vi "MenuSelection(User).vi"(6 "User events":T8, 7 "Clipboard":refnum<vi>, 8 "error in":errorcluster {"code" min=0 max=0}, 10 "ItemTag":string, 11 "Data in":T1={"Class"={"Ants"=refnum, "Layer"=refnum, "Templates"=refnum, "Icon"=refnum, "Glyph"=refnum, "Settings"=refnum, "Tools"=refnum, "History"=refnum}, "Ref"={"Add Layer"=refnum, "Remove Layer"=refnum, "Line Text"=[], "Body Text Spec"=refnum, "DNL_Font"=refnum, "glyph path str"=refnum, "templates path str"=refnum, "Arrow Up"=refnum, "Arrow Down"=refnum, "IE VI Ref"=refnum, "Glyphs tree"=refnum, "Templates tree"=refnum, "Layer Icon Text"=refnum, "Layer Template"=refnum, "Body Text"=refnum, "Search Templates"=refnum, "TextMarker"=refnum, "Tab Control"=refnum, "Search Glyphs"=refnum, "Line Color"=refnum, "DNL_Glyphs []"=refnum, "Fill Color"=refnum, "Tools"=refnum, "Icon"=refnum, "Preview"=refnum, "Ants"=refnum, "Terminals"=refnum, "menu reference"=refnum, "LayerNames"=[], "GlyphLoadAnimation"=refnum, "TemplateLoadAnimation"=refnum, "refreshGlyphs"=refnum, "refreshTemplates"=refnum}, "Support"={"AntsRect"={"left"=0, "top"=0, "right"=0, "bottom"=0}, "Mouse Move Coords"={"Horizontal"=0, "Vertical"=0}, "Mouse Down Coords"={"Horizontal"=0, "Vertical"=0}, "Temp Coord"={"Horizontal"=0, "Vertical"=0}, "Action"=enum."Default", "Edge Color"=4914962, "Fill Color"=16860, "Mouse Down?"=FALSE, "Draft Mode?"=FALSE, "Temp Icon"=bytes[3102], "CTRL Pressed"=FALSE, "Move Selection?"=FALSE, "AntsRect Orig"={"left"=0, "top"=0, "right"=0, "bottom"=0}, "Text"="", "TM Set?"=FALSE, "Mouse inside icon?"=FALSE, "Tool (old value)"=0, "Pencil Move Color"=0, "Swap Colors?"=FALSE, "Shift pressed?"=FALSE}}) -> (0 "error out":errorcluster {"code" min=0 max=0}, 3 "Data out":T1={"Class"={"Ants"=refnum, "Layer"=refnum, "Templates"=refnum, "Icon"=refnum, "Glyph"=refnum, "Settings"=refnum, "Tools"=refnum, "History"=refnum}, "Ref"={"Add Layer"=refnum, "Remove Layer"=refnum, "Line Text"=[], "Body Text Spec"=refnum, "DNL_Font"=refnum, "glyph path str"=refnum, "templates path str"=refnum, "Arrow Up"=refnum, "Arrow Down"=refnum, "IE VI Ref"=refnum, "Glyphs tree"=refnum, "Templates tree"=refnum, "Layer Icon Text"=refnum, "Layer Template"=refnum, "Body Text"=refnum, "Search Templates"=refnum, "TextMarker"=refnum, "Tab Control"=refnum, "Search Glyphs"=refnum, "Line Color"=refnum, "DNL_Glyphs []"=refnum, "Fill Color"=refnum, "Tools"=refnum, "Icon"=refnum, "Preview"=refnum, "Ants"=refnum, "Terminals"=refnum, "menu reference"=refnum, "LayerNames"=[], "GlyphLoadAnimation"=refnum, "TemplateLoadAnimation"=refnum, "refreshGlyphs"=refnum, "refreshTemplates"=refnum}, "Support"={"AntsRect"={"left"=0, "top"=0, "right"=0, "bottom"=0}, "Mouse Move Coords"={"Horizontal"=0, "Vertical"=0}, "Mouse Down Coords"={"Horizontal"=0, "Vertical"=0}, "Temp Coord"={"Horizontal"=0, "Vertical"=0}, "Action"=enum."Default", "Edge Color"=4914962, "Fill Color"=16860, "Mouse Down?"=FALSE, "Draft Mode?"=FALSE, "Temp Icon"=bytes[3102], "CTRL Pressed"=FALSE, "Move Selection?"=FALSE, "AntsRect Orig"={"left"=0, "top"=0, "right"=0, "bottom"=0}, "Text"="", "TM Set?"=FALSE, "Mouse inside icon?"=FALSE, "Tool (old value)"=0, "Pencil Move Color"=0, "Swap Colors?"=FALSE, "Shift pressed?"=FALSE}})   [LabVIEW 2020]
uses:
  Class/Ants/Ants.lvclass
  Class/FakedArray/FakedArray.lvclass
  vi.lib/LabVIEW Icon API/lv_icon/Classes/Icon/Icon.lvclass
  Class/Icon Library/Glyph.lvclass
  Class/Settings/Settings.lvclass
  Class/Tools/Tools Paint.lvclass
  History/History/History.lvclass
  vi.lib/LabVIEW Icon API/lv_icon/Classes/Icon Framework/Icon Framework.lvclass
  vi.lib/LabVIEW Icon API/lv_icon/Classes/Layer/Layer.lvclass
  vi.lib/LabVIEW Icon API/lv_icon/Controls/Layer.ctl
  Controls/Tools.ctl
  lv_icon.lvlib
  vi.lib/LabVIEW Icon API/lv_icon/Controls/Pathes.ctl
  History/History.lvlib
  vi.lib/LabVIEW Icon API/lv_icon/Controls/Graphic.ctl
  <vilib>/Utility/miscctls.llb/LVSelectionTypeDef.ctl
  History/State.ctl
  <vilib>/Utility/miscctls.llb/LVPoint32TypeDef.ctl
  Controls/SupportClass_Action.ctl
  vi.lib/LabVIEW Icon API/lv_icon/Controls/IEColor.ctl
  Controls/Support Cluster.ctl
  Controls/References Cluster.ctl
  Controls/IE Classes.ctl
  Controls/Global Data.ctl
panel:
  in  "Layer name":string="Clipboard"
  in  "glyph":string="Glyph name"
  in  "template":string="Template name"
  in  "Prompt":string="Save Glyph"
  in  "prompt":string="Save Icon Template"
  in  "LayerName":string="Merged Layers"
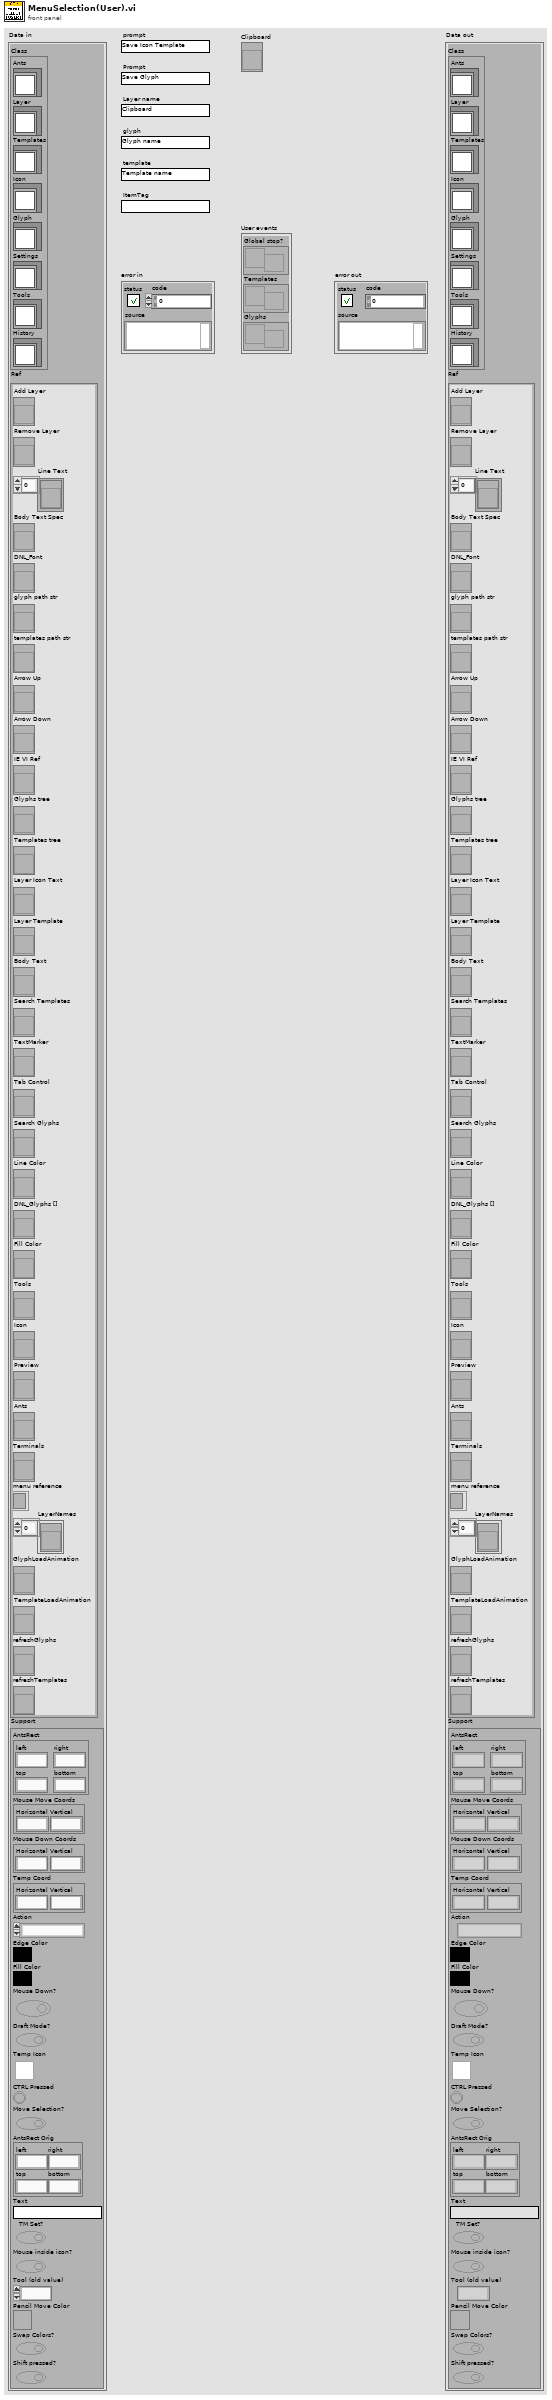
[diagram p1: front panel]
types:
  T1 = typedef "lv_icon.lvlib/Global Data.ctl" = cluster{"Class":T2, "Ref":T3, "Support":T4}
  T2 = typedef "lv_icon.lvlib/IE Classes.ctl" = cluster{"Ants":refnum<class "Ants.lvclass">, "Layer":refnum<class "FakedArray.lvclass">, "Templates":refnum<class "FakedArray.lvclass">, "Icon":refnum<class "Icon.lvclass">, "Glyph":refnum<class "Glyph.lvclass">, "Settings":refnum<class "Settings.lvclass">, "Tools":refnum<class "Tools Paint.lvclass">, "History":refnum<class "History.lvclass">}
  T3 = typedef "lv_icon.lvlib/References Cluster.ctl" = cluster{"Add Layer":refnum<vi>, "Remove Layer":refnum<vi>, "Line Text":refnum<vi>[], "Body Text Spec":refnum<vi>, "DNL_Font":refnum<vi>, "glyph path str":refnum<vi>, "templates path str":refnum<vi>, "Arrow Up":refnum<vi>, "Arrow Down":refnum<vi>, "IE VI Ref":refnum<vi>, "Glyphs tree":refnum<vi>, "Templates tree":refnum<vi>, "Layer Icon Text":refnum<vi>, "Layer Template":refnum<vi>, "Body Text":refnum<vi>, "Search Templates":refnum<vi>, "TextMarker":refnum<vi>, "Tab Control":refnum<vi>, "Search Glyphs":refnum<vi>, "Line Color":refnum<vi>, "DNL_Glyphs []":refnum<vi>, "Fill Color":refnum<vi>, "Tools":refnum<vi>, "Icon":refnum<vi>, "Preview":refnum<vi>, "Ants":refnum<vi>, "Terminals":refnum<vi>, "menu reference":refnum<k9>, "LayerNames":refnum<vi>[], "GlyphLoadAnimation":refnum<vi>, "TemplateLoadAnimation":refnum<vi>, "refreshGlyphs":refnum<vi>, "refreshTemplates":refnum<vi>}
  T4 = typedef "lv_icon.lvlib/Support Cluster.ctl" = cluster{"AntsRect":cluster{"left":i16, "top":i16, "right":i16, "bottom":i16}, "Mouse Move Coords":T5, "Mouse Down Coords":T5, "Temp Coord":T5, "Action":T6, "Edge Color":T7, "Fill Color":T7, "Mouse Down?":bool, "Draft Mode?":bool, "Temp Icon":picture, "CTRL Pressed":bool, "Move Selection?":bool, "AntsRect Orig":cluster{"left":i16, "top":i16, "right":i16, "bottom":i16}, "Text":string, "TM Set?":bool, "Mouse inside icon?":bool, "Tool (old value)":u32, "Pencil Move Color":u32, "Swap Colors?":bool, "Shift pressed?":bool}
  T5 = typedef "LVPoint32TypeDef.ctl" = cluster{"Horizontal":i32, "Vertical":i32}
  T6 = typedef "SupportClass_Action.ctl" = enum16{"Default", "Move Selection", "Glyph Library", "Tool"}
  T7 = typedef "IEColor.ctl" = u32
  T8 = cluster{"Global stop?":refnum<user-event>, "Templates":refnum<user-event>, "Glyphs":refnum<user-event>}
  T9 = typedef "Pathes.ctl" = enum16{"Root Path", "Icon Templates", "Icon Templates VI", "Icon Templates Lib", "Glyphs"}
  T10 = typedef "Graphic.ctl" = cluster{"Rectangle":cluster{"left":i16, "top":i16, "right":i16, "bottom":i16}, "Path":path, "Image":picture, "Filter":string, "FileName":string}
  T11 = typedef "Layer.ctl" = cluster{"LayerIcon":picture, "LayerName":string, "Opacity":u8, "Visibility?":bool}
  T12 = typedef "lv_icon.lvlib/History.lvlib/State.ctl" = cluster{"Template":string, "Layers":string, "Body Text":string, "Icon Text Layer":string, "Template Layer":string, "Templates Search":string, "Glyphs Search":string}
  T13 = enum32{"Pencil", "Line", "Dropper", "Fill", "Rectangle", "Filled Rectangle", "Ellipse", "Filled Ellipse", "Eraser", "Text", "Select", "Move"}
  T14 = typedef "LVSelectionTypeDef.ctl" = cluster{"Selection Start":u32, "Selection End":u32}
  T15 = typedef "Tools.ctl" = enum32{"Pencil", "Line", "Dropper", "Fill", "Rectangle", "Filled Rectangle", "Ellipse", "Filled Ellipse", "Eraser", "Text", "Select", "Move"}
  T16 = typedef "imagedata.ctl" = cluster{"image type":i32, "image depth":i32, "image":u8[], "mask":u8[], "colors":u32[], "Rectangle":cluster{"left":i16, "top":i16, "right":i16, "bottom":i16}}
  T17 = typedef "Font.ctl" = string
  T18 = typedef "Alignment.ctl" = u16
  T19 = typedef "Font Size.ctl" = u8
  T20 = cluster{"Line 1 text":string, "Line 2 text":string, "Line 3 text":string, "Line 4 text":string, "Line 1 color":u32, "Line 2 color":u32, "Line 3 color":u32, "Line 4 color":u32, "Body Text Spec":cluster{"DNL_Font":T17, "Alignment":T18, "Size":T19}, "Center text vertically":bool, "Capitalize Text":bool}
  T21 = cluster{"left":i16, "top":i16, "right":i16, "bottom":i16}
  T22 = cluster{"Horizontal":i32, "Vertical":i32, "Vertical 2":i32, "Vertical 3":i32}
  T23 = cluster{"Left":i32, "Top":i32, "Right":i32, "Bottom":i32}
  T24 = typedef "Icon Editor Invoker Type.ctl" = enum32{"Unknown Icon Source", "VI Icon", "Library Icon (any library type)", "Palette icon", "Icon from App Method"}
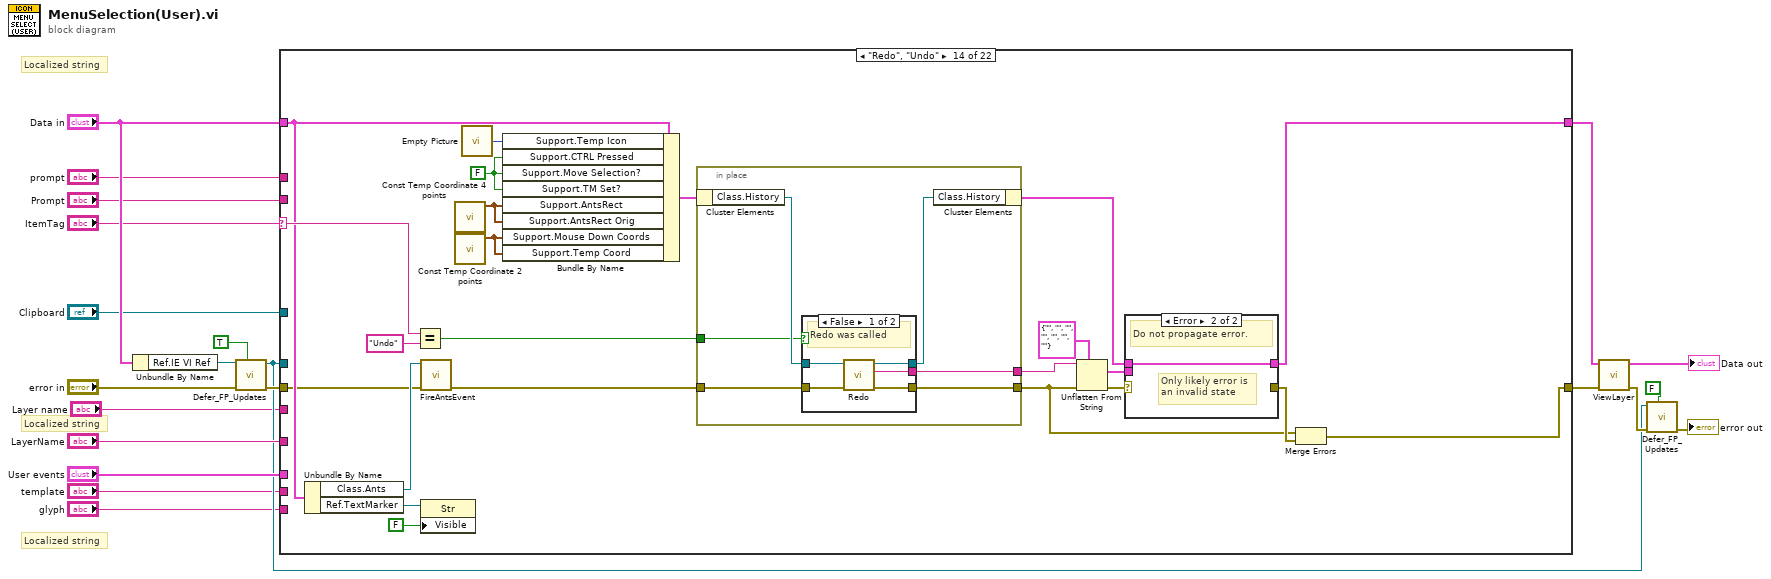
[diagram p0: block diagram]
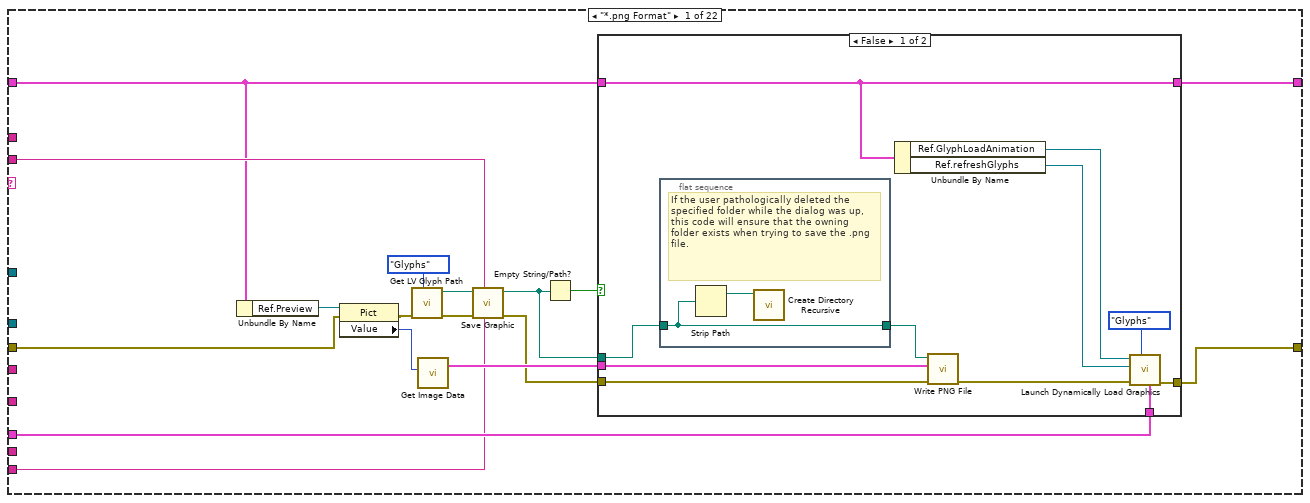
[diagram p2: hidden frame]
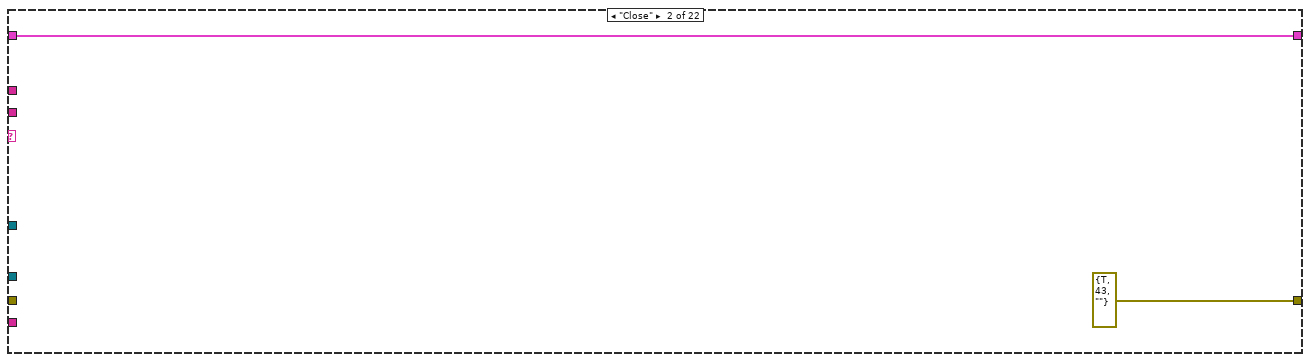
[diagram p4: hidden frame]
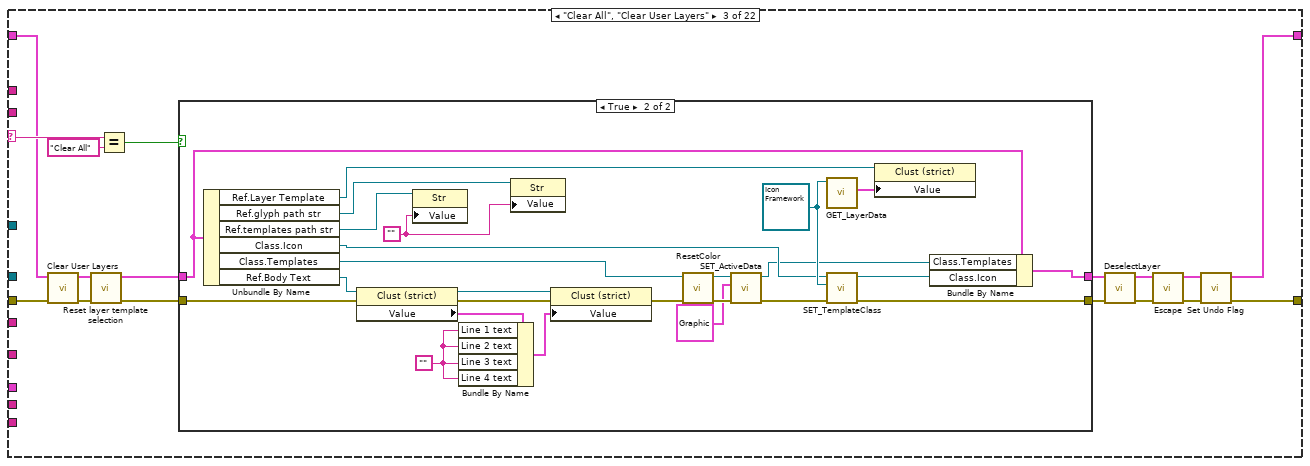
[diagram p5: hidden frame]
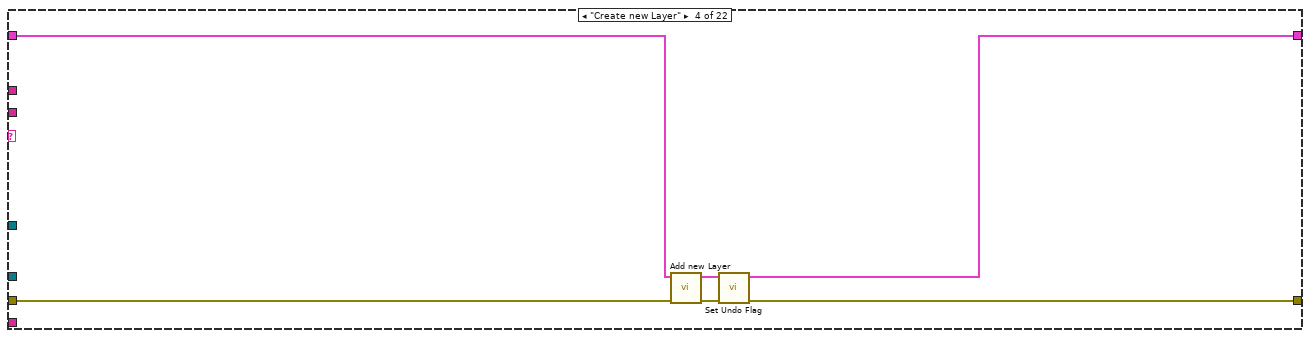
[diagram p7: hidden frame]
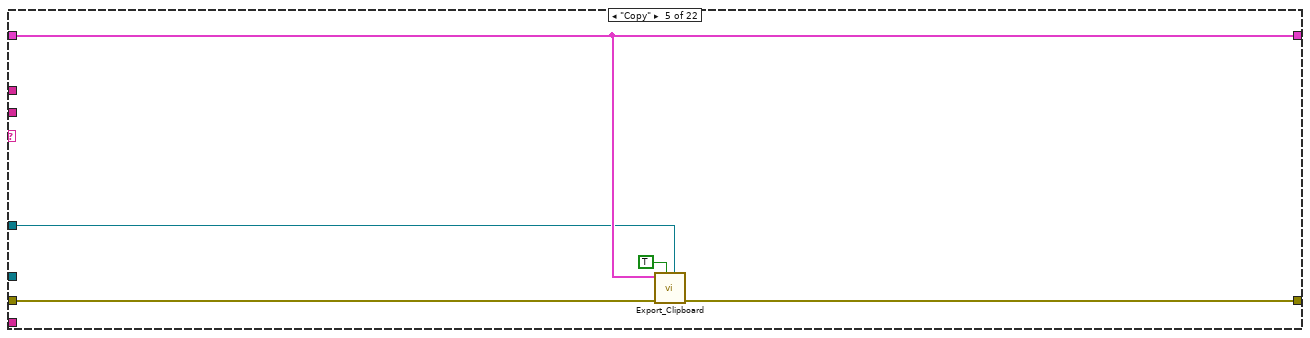
[diagram p8: hidden frame]
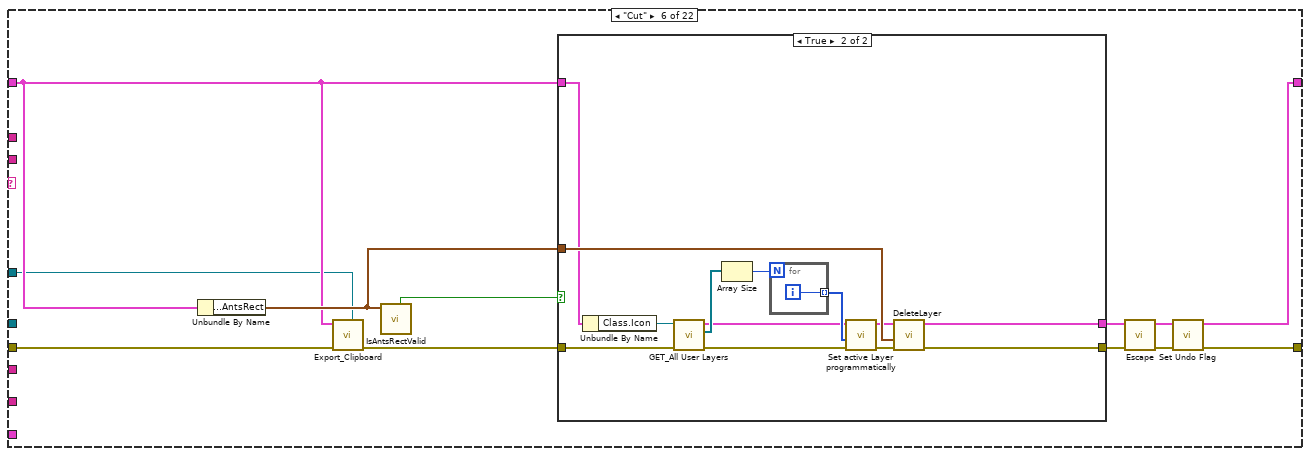
[diagram p9: hidden frame]
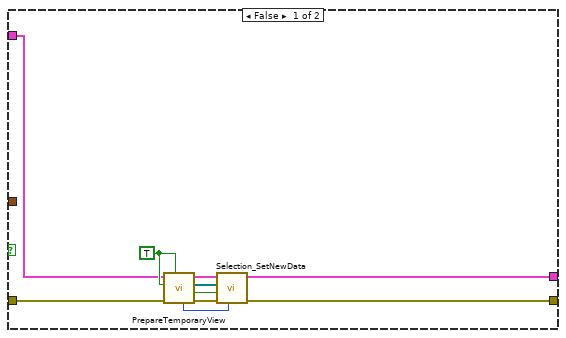
[diagram p10: hidden frame]
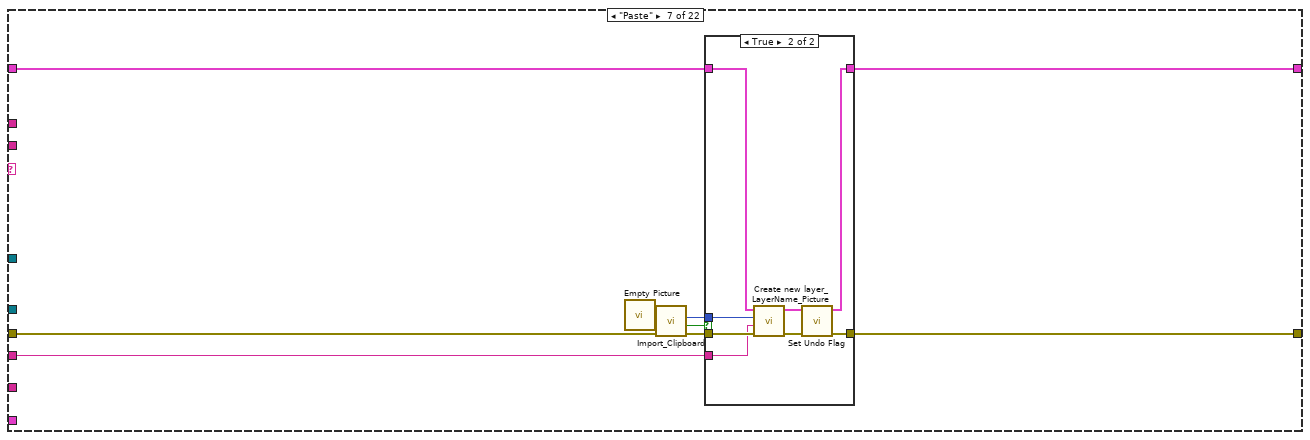
[diagram p11: hidden frame]
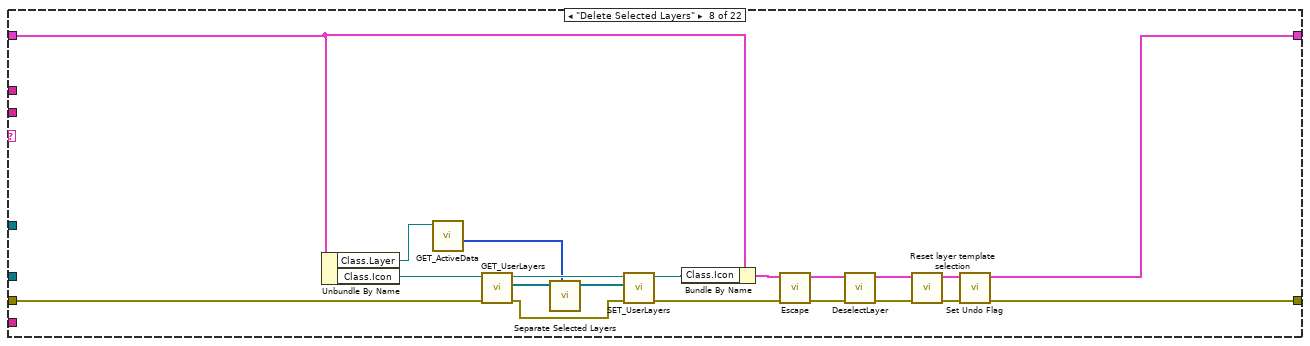
[diagram p13: hidden frame]
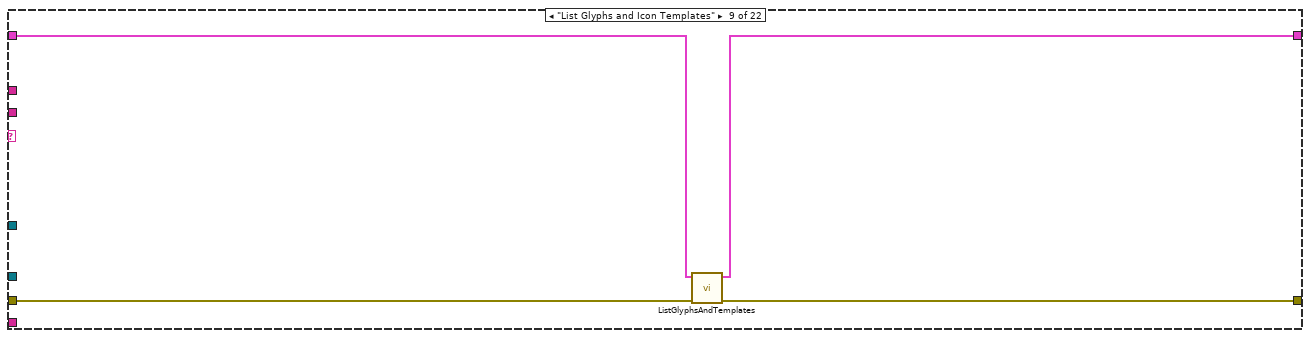
[diagram p14: hidden frame]
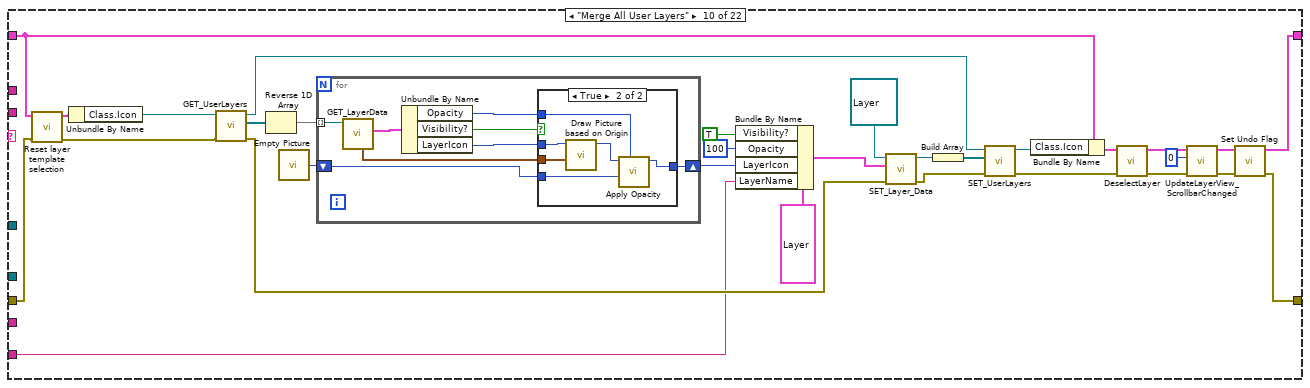
[diagram p15: hidden frame]
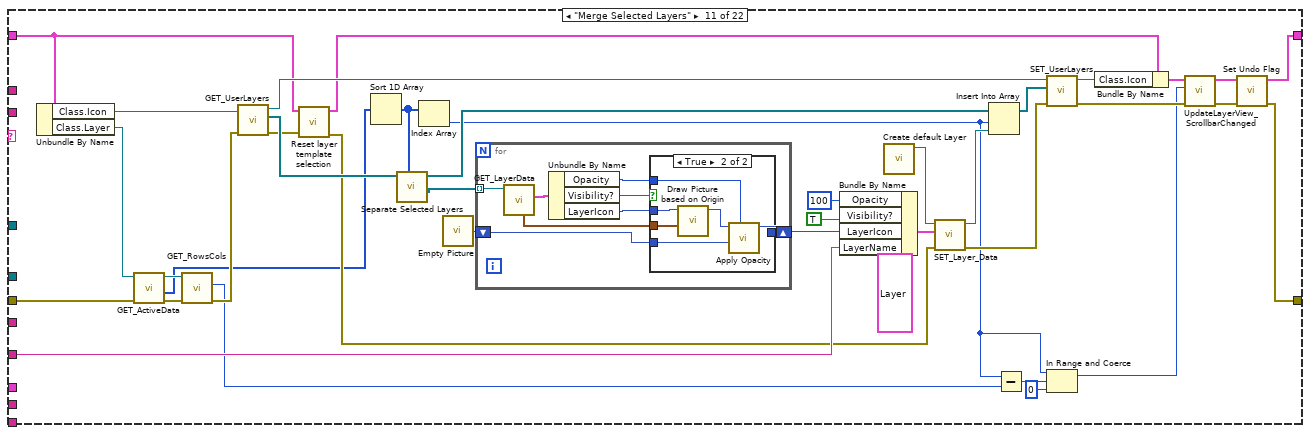
[diagram p17: hidden frame]
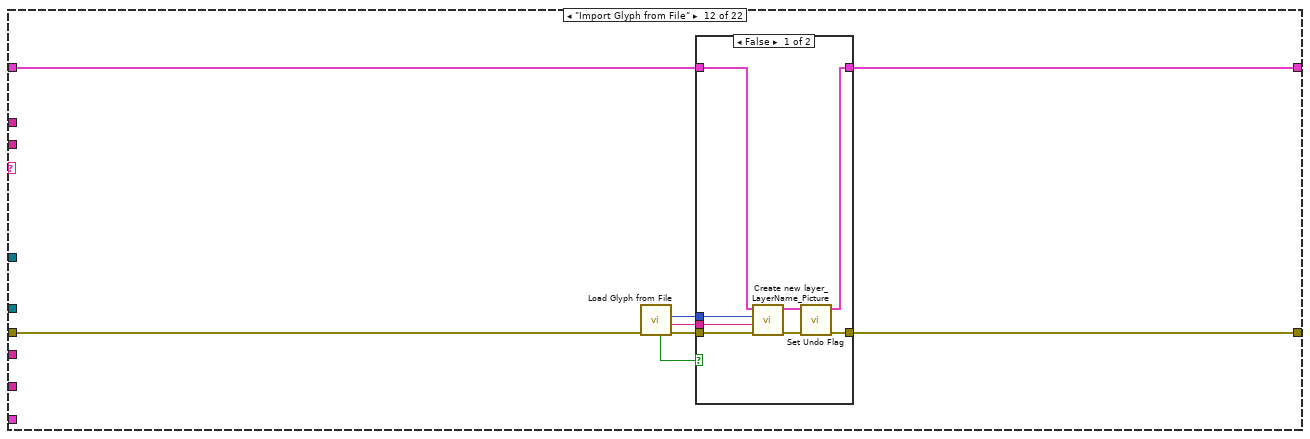
[diagram p19: hidden frame]
diagram:
  # "Localized string"
  # "Localized string"
  # "Localized string"
  n1 = Unbundle By Name("Data in") -> ("Ref.IE VI Ref"=w9:refnum<vi>)
  n2 = call "Defer_FP_Updates.vi"("Defer Panel Updates"=TRUE, "error in"="error in", "lv_icon.vi in"=w9) -> ("error out"=w11:errorcluster, "lv icon.vi out"=w5:refnum<vi>)  [unwired: 7 out]
  n3 = case shown="\"Redo\", \"Undo\"" "ItemTag" {
    selector: "ItemTag" -> [_ _ w72 _ _ _ _ _ _ _ _ _ _ w335 _ w416 _ _ _ _ _ _]
    tunnel: w11 -> [w26 _ w63 w103 w110 w117 w150 w177 w188 w205 w238 w292 w319 w331 w375 w407 w424 w426 w448 w470 w500 w505]
    tunnel: [w27 errorcluster {"status"=TRUE, "code"=43, "source"=""} ("Icon 43") w58 w102 w109 w113 w153 w167 w187 w191 w236 w294 w306 w320 w373 w409 w418 w427 w454 w469 w501 w505] -> w15
    tunnel: "LayerName" -> [_ _ _ _ _ _ _ _ _ w206 w261 _ _ _ _ _ _ _ _ _ _ _]
    tunnel: "prompt" -> [_ _ _ _ _ _ _ _ _ _ _ _ _ _ _ _ _ _ _ w472 _ _]
    tunnel: "Prompt" -> [w28 _ _ _ _ _ _ _ _ _ _ _ _ _ _ _ _ _ _ _ _ _]
    tunnel: "User events" -> [w33 _ _ _ _ _ _ _ _ _ _ _ _ _ _ _ _ _ w453 w478 _ _]
    tunnel: [w22 w54 w56 w100 w107 w111 w152 w165 w185 w189 w234 w293 w308 w330 w374 w408 w417 w425 w439 w465 w499 w504] -> w13
    tunnel: "Data in" -> [w23 w54 w64 w105 w107 w115 w154 w172 w186 w201 w254 w295 w311 w333 w370 w410 w423 w430 w440 w475 w499 w504]
    tunnel: w5 -> [_ _ _ _ _ _ _ _ _ _ _ _ _ _ _ _ _ _ _ _ w503 _]
    tunnel: "template" -> [_ _ _ _ _ _ _ _ _ _ _ _ _ _ _ _ _ _ _ w467 _ _]
    tunnel: "glyph" -> [w24 _ _ _ _ _ _ _ _ _ _ _ _ _ _ _ _ _ _ _ _ _]
    tunnel: "Layer name" -> [_ _ _ _ _ _ w146 _ _ _ _ _ _ _ _ _ _ _ _ _ _ _]
    tunnel: "Clipboard" -> [_ _ _ _ w106 w114 _ _ _ _ _ _ _ _ _ _ _ _ _ _ _ _]
    frame "*.png Format" {
      n4 = Unbundle By Name(w23) -> ("Ref.Preview"=w38:refnum<vi>)
      n5 = property class="Pict"(reference=w38, error in=w26) -> (error out=w34:errorcluster, "Value"=w36:picture)  [unwired: 1 out]
      n6 = call "Get LV Glyph Path.vi"("Path"=Pathes."Glyphs", "error in (no error)"=w34) -> ("error out"=w32:errorcluster, "Requested Path"=w29:path)  [unwired: 1 in, 7 out]
      n7 = call "Get Image Data.vi"("Pic In"=w36) -> ("image data out"=w37:T16)  [unwired: 3 in, 7 out]
      n8 = call "Save Graphic.vi"("Loc string caption"=w24, "FP Title"=w28, "error in (no error)"=w32, "Start path in"=w29) -> ("error out"=w31:errorcluster, "Output"=w30:path)  [unwired: 6 out]
      n9 = Empty String/Path?(string/path=w30) -> (empty?=w25:bool)
      n10 = case shown="False" w25 {
        tunnel: w37 -> [w49 _]
        tunnel: w33 -> [w46 _]
        tunnel: w31 -> [w45 w53]
        tunnel: w30 -> [w40 _]
        tunnel: [w44 w53] -> w27
        tunnel: w23 -> [w43 w52]
        tunnel: [w43 w52] -> w22
        frame False {
          n11 = flat-sequence {
            tunnel: w40 -> [w51]
            tunnel: [w51] -> w39
            frame #0 {
              # "If the user pathologically deleted the specified folder while the dialog was up, this code will ensure that the owning folder exists when trying to save the .png file."
              n12 = Strip Path(path=w51) -> (stripped path=w50:path)  [unwired: 1 out]
              n13 = call <vilib>:"Create Directory Recursive.vi"("directory"=w50) -> ()  [unwired: 4 in, 3 out]
            }
          }
          n14 = Unbundle By Name(w43) -> ("Ref.GlyphLoadAnimation"=w41:refnum<vi>, "Ref.refreshGlyphs"=w42:refnum<vi>)
          n15 = call <vilib>:"Write PNG File.vi"("error in (no error)"=w45, "image data"=w49, "path to PNG file"=w39) -> ("error out"=w48:errorcluster)  [unwired: 1 in, 7 out]
          n16 = call "Launch Dynamically Load Graphics.vi"("User events"=w46, "Path"=Pathes."Glyphs", "error in (no error)"=w48, "button ref"=w42, "animatedDecoration ref"=w41) -> ("error out"=w44:errorcluster)  [unwired: 1 in, 5 out]
        }
        frame True {
        }
      }
    }
    frame "Close" {
    }
    frame "Clear All", "Clear User Layers" {
      n17 = call "Clear User Layers.vi"("error in"=w63, "Data in"=w64) -> ("error out"=w62:errorcluster, "Data out"=w61:T1)  [unwired: 8 out]
      n18 = call "Reset layer template selection.vi"("error in (no error)"=w62, "Data in"=w61) -> ("error out"=w59:errorcluster, "Data out"=w60:T1)  [unwired: 1 in, 7 out]
      n19 = Equal?(x=w72, y="Clear All") -> (x = y?=w71:bool)
      n20 = case shown="True" w71 {
        tunnel: w59 -> [w74 w89]
        tunnel: w60 -> [w73 w81]
        tunnel: [w74 w84] -> w69
        tunnel: [w73 w82] -> w68
        frame False {
        }
        frame True {
          w99 = refnum<class "Icon Framework.lvclass"> refnum ("lv_icon.lvlib:Icon Framework.lvclass")
          w78 = ""
          w94 = ""
          n21 = Unbundle By Name(w81) -> ("Ref.Layer Template"=w76:refnum<vi>, "Ref.glyph path str"=w79:refnum<vi>, "Ref.templates path str"=w80:refnum<vi>, "Class.Icon"=w87:refnum<class "Icon.lvclass">, "Class.Templates"=w88:refnum<class "FakedArray.lvclass">, "Ref.Body Text"=w98:refnum<vi>)
          n22 = property class="Clust (strict)"(reference=w98, error in=w89) -> (reference out=w97:refnum<vi>, error out=w96:errorcluster, "Value"=w95:T20)
          n23 = property class="Str"(reference=w80, "Value"=w78) -> ()  [unwired: 1 in, 2 out]
          n24 = Bundle By Name(cluster=w95, "Line 1 text"=w94, "Line 2 text"=w94, "Line 3 text"=w94, "Line 4 text"=w94) -> (w90:T20)
          n25 = property class="Str"(reference=w79, "Value"=w78) -> ()  [unwired: 1 in, 2 out]
          n26 = property class="Clust (strict)"(reference=w97, error in=w96, "Value"=w90) -> (error out=w77:errorcluster)  [unwired: 1 out]
          n27 = call "ResetColor.vi"("error in (no error)"=w77, "FakedArray in"=w88) -> ("error out"=w92:errorcluster, "FakedArray out"=w93:refnum<class "FakedArray.lvclass">)  [unwired: 8 out]
          n28 = call-dynamic "SET_ActiveData.vi"("error in (no error)"=w92, "Active Data"=T10 {"Rectangle"={"left"=0, "top"=0, "right"=0, "bottom"=0}, "Path"=path "", "Image"=bytes[0], "Filter"="", "FileName"=""} ("Path & Icon"), "FakedArray.lvclass in"=w93) -> ("error out"=w86:errorcluster, "FakedArray.lvclass out"=w83:refnum<class "FakedArray.lvclass">)  [unwired: 7 out]
          n29 = call-dynamic "GET_LayerData.vi"("Layer.lvclass in"=w99) -> ("Data"=w75:T11)  [unwired: 1 in, 9 out]
          n30 = call-dynamic "SET_TemplateClass.vi"("error in (no error)"=w86, "Icon Framework.lvclass"=w99, "Icon.lvclass in"=w87) -> ("error out"=w84:errorcluster, "Icon.lvclass out"=w85:refnum<class "Icon.lvclass">)  [unwired: 7 out]
          n31 = property class="Clust (strict)"(reference=w76, "Value"=w75) -> ()  [unwired: 1 in, 2 out]
          n32 = Bundle By Name(cluster=w81, "Class.Templates"=w83, "Class.Icon"=w85) -> (w82:T1)
        }
      }
      n33 = call "DeselectLayer.vi"("error in (no error)"=w69, "Data in"=w68) -> ("error out"=w65:errorcluster, "Data out"=w67:T1)  [unwired: 8 out]
      n34 = call "Escape.vi"("error in"=w65, "Data in"=w67) -> ("error out"=w66:errorcluster, "Data out"=w57:T1)  [unwired: 2 in, 6 out]
      n35 = call "Set Undo Flag.vi"("error in"=w66, "Data in"=w57) -> ("error out"=w58:errorcluster, "Data out"=w56:T1)  [unwired: 8 in]
    }
    frame "Create new Layer" {
      n36 = call "Add new Layer.vi"("error in"=w103, "Data in"=w105) -> ("error out"=w104:errorcluster, "Data out"=w101:T1)  [unwired: 8 out]
      n37 = call "Set Undo Flag.vi"("error in"=w104, "Data in"=w101) -> ("error out"=w102:errorcluster, "Data out"=w100:T1)  [unwired: 8 in]
    }
    frame "Copy" {
      n38 = call "Export_Clipboard.vi"("Clipboard"=w106, "Is Copy? (F)"=TRUE, "error in"=w110, "Data in"=w107) -> ("error out"=w109:errorcluster)  [unwired: 1 in, 6 out]
    }
    frame "Cut" {
      n39 = Unbundle By Name(w115) -> ("Support.AntsRect"=w119:T21)
      n40 = call "Export_Clipboard.vi"("Clipboard"=w114, "error in"=w117, "Data in"=w115) -> ("error out"=w120:errorcluster)  [unwired: 1 in, 7 out]
      n41 = call "IsAntsRectValid.vi"("AntsRect"=w119) -> ("Max. Rect size?"=w121:bool)  [unwired: 10 out]
      n42 = case shown="True" w121 {
        tunnel: [w132 w143] -> w116
        tunnel: [w131 w144] -> w118
        tunnel: w120 -> [w124 w135]
        tunnel: w119 -> [_ w142]
        tunnel: w115 -> [w123 w133]
        frame False {
          w130 = TRUE ("Delete Selected Area?")
          n43 = call "PrepareTemporaryView.vi"("Delete Selected Area?"=w130, "error in (no error)"=w124, "Valid Selection?"=w130, "Data in"=w123) -> ("error out"=w127:errorcluster, "Highlighted?"=w128:bool, "All Layers out"=w129:refnum<class "Layer.lvclass">[], "Data out"=w125:T1, "#Active Layer"=w126:i32)  [unwired: 1 in, 2 out]
          n44 = call "Selection_SetNewData.vi"("#Active Layer"=w126, "error in"=w127, "Highlighted?"=w128, "All Layers In"=w129, "Data in"=w125) -> ("error out"=w132:errorcluster, "Data out"=w131:T1)  [unwired: 1 in, 3 out]
        }
        frame True {
          n45 = Unbundle By Name(w133) -> ("Class.Icon"=w141:refnum<class "Icon.lvclass">)
          n46 = call-dynamic "GET_All User Layers.vi"("error in (no error)"=w135, "Icon.lvclass in"=w141) -> ("error out"=w140:errorcluster, "User Layer"=w137:refnum<class "Layer.lvclass">[])  [unwired: 7 in, 1 out]
          n47 = Array Size(array=w137) -> (size(s)=w138:i32)
          n48 = for {
            N: w138 -> [_]
            tunnel: [w145] -> w139 mode=indexing
            i -> [w145]
          }
          n49 = call "Set active Layer programmatically.vi"("error in"=w140, "Active Layer []"=w139, "Data in"=w133) -> ("error out"=w134:errorcluster, "Data out"=w136:T1)  [unwired: 7 in]
          n50 = call "DeleteLayer.vi"("error in"=w134, "AntsRect"=w142, "Data in"=w136) -> ("error out"=w143:errorcluster, "Data out"=w144:T1)  [unwired: 5 out]
        }
      }
      n51 = call "Escape.vi"("error in"=w116, "Data in"=w118) -> ("error out"=w122:errorcluster, "Data out"=w112:T1)  [unwired: 2 in, 6 out]
      n52 = call "Set Undo Flag.vi"("error in"=w122, "Data in"=w112) -> ("error out"=w113:errorcluster, "Data out"=w111:T1)  [unwired: 8 in]
    }
    frame "Paste" {
      n53 = call "Empty Picture"() -> ("empty picture"=w151:picture)
      n54 = call "Import_Clipboard.vi"("error in (no error)"=w150, "Picture in"=w151) -> ("error out"=w149:errorcluster, "Valid?"=w148:bool, "Picture"=w147:picture)  [unwired: 1 in, 6 out]
      n55 = case shown="True" w148 {
        tunnel: w154 -> [w155 w164]
        tunnel: [w156 w159] -> w153
        tunnel: [w155 w157] -> w152
        tunnel: w149 -> [w156 w162]
        tunnel: w147 -> [_ w161]
        tunnel: w146 -> [_ w160]
        frame False {
        }
        frame True {
          n56 = call "Create new layer_LayerName_Picture.vi"("error in"=w162, "Layer name"=w160, "Picture"=w161, "Data in"=w164) -> ("error out"=w163:errorcluster, "Data out"=w158:T1)  [unwired: 6 in]
          n57 = call "Set Undo Flag.vi"("error in"=w163, "Data in"=w158) -> ("error out"=w159:errorcluster, "Data out"=w157:T1)  [unwired: 8 in]
        }
      }
    }
    frame "Delete Selected Layers" {
      n58 = Unbundle By Name(w172) -> ("Class.Layer"=w170:refnum<class "FakedArray.lvclass">, "Class.Icon"=w180:refnum<class "Icon.lvclass">)
      n59 = call-dynamic "GET_ActiveData.vi"("FakedArray in"=w170) -> ("Active Data []"=w178:i32[])  [unwired: 1 in, 9 out]
      n60 = call-dynamic "GET_UserLayers.vi"("error in (no error)"=w177, "Icon.lvclass in"=w180) -> ("error out"=w181:errorcluster, "All Layers"=w184:refnum<class "Layer.lvclass">[], "Icon.lvclass out"=w183:refnum<class "Icon.lvclass">)  [unwired: 7 out]
      n61 = call "Separate Selected Layers.vi"("Active Indices"=w178, "All Layers"=w184) -> ("Layers out not in Array"=w182:refnum<class "Layer.lvclass">[])  [unwired: 9 out]
      n62 = call-dynamic "SET_UserLayers.vi"("error in"=w181, "Layers"=w182, "Icon.lvclass in"=w183) -> ("error out"=w169:errorcluster, "Icon.lvclass out"=w179:refnum<class "Icon.lvclass">)  [unwired: 7 in]
      n63 = Bundle By Name(cluster=w172, "Class.Icon"=w179) -> (w171:T1)
      n64 = call "Escape.vi"("error in"=w169, "Data in"=w171) -> ("error out"=w176:errorcluster, "Data out"=w175:T1)  [unwired: 8 out]
      n65 = call "DeselectLayer.vi"("error in (no error)"=w176, "Data in"=w175) -> ("error out"=w173:errorcluster, "Data out"=w174:T1)  [unwired: 8 out]
      n66 = call "Reset layer template selection.vi"("error in (no error)"=w173, "Data in"=w174) -> ("error out"=w168:errorcluster, "Data out"=w166:T1)  [unwired: 1 in, 7 out]
      n67 = call "Set Undo Flag.vi"("error in"=w168, "Data in"=w166) -> ("error out"=w167:errorcluster, "Data out"=w165:T1)  [unwired: 8 in]
    }
    frame "List Glyphs and Icon Templates" {
      n68 = call "ListGlyphsAndTemplates.vi"("error in"=w188, "Data in"=w186) -> ("error out"=w187:errorcluster, "Data out"=w185:T1)  [unwired: 8 out]
    }
    frame "Merge All User Layers" {
      n69 = call "Reset layer template selection.vi"("error in (no error)"=w205, "Data in"=w201) -> ("error out"=w204:errorcluster, "Data out"=w203:T1)  [unwired: 1 in, 7 out]
      n70 = Unbundle By Name(w203) -> ("Class.Icon"=w202:refnum<class "Icon.lvclass">)
      n71 = call-dynamic "GET_UserLayers.vi"("error in (no error)"=w204, "Icon.lvclass in"=w202) -> ("error out"=w210:errorcluster, "All Layers"=w218:refnum<class "Layer.lvclass">[], "Icon.lvclass out"=w217:refnum<class "Icon.lvclass">)  [unwired: 7 out]
      n72 = Reverse 1D Array(array=w218) -> (reversed array=w208:refnum<class "Layer.lvclass">[])
      n73 = call "Empty Picture"() -> ("empty picture"=w207:picture)
      n74 = for {
        shift-right: [w223] -> w214
        shift-left: w207 -> [w224]
        tunnel: w208 -> [w219] mode=indexing
        n75 = call-dynamic "GET_LayerData.vi"("Layer.lvclass in"=w219) -> ("Data"=w221:T11, "Origin"=w220:T5)  [unwired: 1 in, 8 out]
        n76 = Unbundle By Name(w221) -> ("Opacity"=w225:u8, "Visibility?"=w226:bool, "LayerIcon"=w222:picture)
        n77 = case shown="True" w226 {
          tunnel: w225 -> [_ w233]
          tunnel: w224 -> [w227 w232]
          tunnel: [w227 w231] -> w223
          tunnel: w222 -> [_ w230]
          tunnel: w220 -> [_ w229]
          frame False {
          }
          frame True {
            n78 = call "Draw Picture based on Origin.vi"("Origin"=w229, "LayerIcon in"=w230) -> ("LayerIcon out"=w228:picture)  [unwired: 1 in, 8 out]
            n79 = call "Apply Opacity.vi"("% (100)"=w233, "Bottom"=w232, "Top"=w228) -> ("new picture"=w231:picture)  [unwired: 8 out]
          }
        }
      }
      n80 = Bundle By Name(cluster=T11 {"LayerIcon"=bytes[0], "LayerName"="", "Opacity"=0, "Visibility?"=FALSE} ("Data"), "Visibility?"=TRUE, "Opacity"=u8 100, "LayerIcon"=w214, "LayerName"=w206) -> (w213:T11)
      n81 = call-dynamic "SET_Layer_Data.vi"("error in (no error)"=w210, "Data"=w213, "Layer.lvclass in"=refnum<class "Layer.lvclass"> refnum) -> ("error out"=w211:errorcluster, "Layer.lvclass out"=w216:refnum<class "Layer.lvclass">)  [unwired: 1 in, 6 out]
      n82 = Build Array(w216) -> (w209:refnum<class "Layer.lvclass">[])
      n83 = call-dynamic "SET_UserLayers.vi"("error in"=w211, "Layers"=w209, "Icon.lvclass in"=w217) -> ("error out"=w199:errorcluster, "Icon.lvclass out"=w200:refnum<class "Icon.lvclass">)  [unwired: 7 in]
      n84 = Bundle By Name(cluster=w201, "Class.Icon"=w200) -> (w198:T1)
      n85 = call "DeselectLayer.vi"("error in (no error)"=w199, "Data in"=w198) -> ("error out"=w194:errorcluster, "Data out"=w195:T1)  [unwired: 8 out]
      n86 = call "UpdateLayerView_ScrollbarChanged.vi"("error in"=w194, "Scrollbar Position"=0, "Data in"=w195) -> ("error out"=w193:errorcluster, "Data out"=w190:T1)  [unwired: 7 out]
      n87 = call "Set Undo Flag.vi"("error in"=w193, "Data in"=w190) -> ("error out"=w191:errorcluster, "Data out"=w189:T1)  [unwired: 8 in]
    }
    frame "Merge Selected Layers" {
      n88 = Unbundle By Name(w254) -> ("Class.Icon"=w256:refnum<class "Icon.lvclass">, "Class.Layer"=w241:refnum<class "FakedArray.lvclass">)
      n89 = call-dynamic "GET_ActiveData.vi"("error in (no error)"=w238, "FakedArray in"=w241) -> ("error out"=w239:errorcluster, "Active Data []"=w237:i32[], "FakedArray out"=w240:refnum<class "FakedArray.lvclass">)  [unwired: 7 out]
      n90 = call-dynamic "GET_RowsCols.vi"("error in (no error)"=w239, "FakedArray.lvclass in"=w240) -> ("error out"=w249:errorcluster, "# Rows"=w248:i32)  [unwired: 8 out]
      n91 = call-dynamic "GET_UserLayers.vi"("error in (no error)"=w249, "Icon.lvclass in"=w256) -> ("error out"=w260:errorcluster, "All Layers"=w265:refnum<class "Layer.lvclass">[], "Icon.lvclass out"=w266:refnum<class "Icon.lvclass">)  [unwired: 7 out]
      n92 = call "Reset layer template selection.vi"("error in (no error)"=w260, "Data in"=w254) -> ("error out"=w259:errorcluster, "Data out"=w253:T1)  [unwired: 1 in, 7 out]
      n93 = Sort 1D Array(array=w237) -> (sorted array=w272:i32[])
      n94 = call "Separate Selected Layers.vi"("Active Indices"=w272, "All Layers"=w265) -> ("Layers out in Array"=w263:refnum<class "Layer.lvclass">[], "Layers out not in Array"=w264:refnum<class "Layer.lvclass">[])  [unwired: 8 out]
      n95 = Index Array(array=w272) -> (element=w246:i32)  [unwired: 1 in]
      n96 = call "Empty Picture"() -> ("empty picture"=w268:picture)
      n97 = for {
        shift-right: [w277] -> w270
        shift-left: w268 -> [w278]
        tunnel: w263 -> [w273] mode=indexing
        n98 = call-dynamic "GET_LayerData.vi"("Layer.lvclass in"=w273) -> ("Data"=w275:T11, "Origin"=w274:T5)  [unwired: 1 in, 8 out]
        n99 = Unbundle By Name(w275) -> ("Opacity"=w279:u8, "Visibility?"=w280:bool, "LayerIcon"=w276:picture)
        n100 = case shown="True" w280 {
          tunnel: w279 -> [_ w287]
          tunnel: w278 -> [w281 w286]
          tunnel: [w281 w285] -> w277
          tunnel: w276 -> [_ w284]
          tunnel: w274 -> [_ w283]
          frame False {
          }
          frame True {
            n101 = call "Draw Picture based on Origin.vi"("Origin"=w283, "LayerIcon in"=w284) -> ("LayerIcon out"=w282:picture)  [unwired: 1 in, 8 out]
            n102 = call "Apply Opacity.vi"("% (100)"=w287, "Bottom"=w286, "Top"=w282) -> ("new picture"=w285:picture)  [unwired: 8 out]
          }
        }
      }
      n103 = Bundle By Name(cluster=T11 {"LayerIcon"=bytes[0], "LayerName"="", "Opacity"=0, "Visibility?"=FALSE} ("Data"), "Opacity"=u8 100, "Visibility?"=TRUE, "LayerIcon"=w270, "LayerName"=w261) -> (w269:T11)
      n104 = call "Create default Layer.vi"() -> ("Layer.lvclass out"=w257:refnum<class "Layer.lvclass">)  [unwired: 1 in, 10 out]
      n105 = call-dynamic "SET_Layer_Data.vi"("error in (no error)"=w259, "Data"=w269, "Layer.lvclass in"=w257) -> ("error out"=w258:errorcluster, "Layer.lvclass out"=w267:refnum<class "Layer.lvclass">)  [unwired: 1 in, 6 out]
      n106 = Insert Into Array(array=w264, index=w246, new element=w267) -> (w262:refnum<class "Layer.lvclass">[])
      n107 = Subtract(x=w246, y=w248) -> (x-y=w247:i32)
      n108 = call-dynamic "SET_UserLayers.vi"("error in"=w258, "Layers"=w262, "Icon.lvclass in"=w266) -> ("error out"=w251:errorcluster, "Icon.lvclass out"=w255:refnum<class "Icon.lvclass">)  [unwired: 7 in]
      n109 = In Range and Coerce(upper limit=w246, x=w247, lower limit=0) -> (coerced(x)=w244:i32)  [unwired: 1 out]
      n110 = Bundle By Name(cluster=w253, "Class.Icon"=w255) -> (w252:T1)
      n111 = call "UpdateLayerView_ScrollbarChanged.vi"("error in"=w251, "Scrollbar Position"=w244, "Data in"=w252) -> ("error out"=w250:errorcluster, "Data out"=w235:T1)  [unwired: 7 out]
      n112 = call "Set Undo Flag.vi"("error in"=w250, "Data in"=w235) -> ("error out"=w236:errorcluster, "Data out"=w234:T1)  [unwired: 8 in]
    }
    frame "Import Glyph from File" {
      n113 = call "Load Glyph from File.vi"("error in (no error)"=w292) -> ("error out"=w291:errorcluster, "file name"=w288:string, "Pic Out"=w289:picture, "Canceled?"=w290:bool)  [unwired: 7 in]
      n114 = case shown="False" w290 {
        tunnel: w295 -> [w301 w304]
        tunnel: [w298 w305] -> w294
        tunnel: [w296 w304] -> w293
        tunnel: w291 -> [w303 w305]
        tunnel: w289 -> [w299 _]
        tunnel: w288 -> [w300 _]
        frame False {
          n115 = call "Create new layer_LayerName_Picture.vi"("error in"=w303, "Layer name"=w300, "Picture"=w299, "Data in"=w301) -> ("error out"=w302:errorcluster, "Data out"=w297:T1)  [unwired: 6 in]
          n116 = call "Set Undo Flag.vi"("error in"=w302, "Data in"=w297) -> ("error out"=w298:errorcluster, "Data out"=w296:T1)  [unwired: 8 in]
        }
        frame True {
        }
      }
    }
    frame "Import Icon from Owning Library" {
      n117 = Unbundle By Name(w311) -> ("Class.Icon"=w318:refnum<class "Icon.lvclass">)
      n118 = call "Read Data from Caller.vi"("error in (no error)"=w319) -> ("error out"=w317:errorcluster, "Library Icon"=w315:picture)  [unwired: 5 in, 4 out]
      n119 = call-dynamic "GET_UserLayers.vi"("error in (no error)"=w317, "Icon.lvclass in"=w318) -> ("error out"=w312:errorcluster, "All Layers"=w316:refnum<class "Layer.lvclass">[], "Icon.lvclass out"=w314:refnum<class "Icon.lvclass">)  [unwired: 7 out]
      n120 = call "Create or Substitute NI_Layer layer.vi"("All Layers in"=w316, "new picture"=w315) -> ("All Layers out"=w313:refnum<class "Layer.lvclass">[])
      n121 = call-dynamic "SET_UserLayers.vi"("error in"=w312, "Layers"=w313, "Icon.lvclass in"=w314) -> ("error out"=w307:errorcluster, "Icon.lvclass out"=w310:refnum<class "Icon.lvclass">)  [unwired: 7 in]
      n122 = Bundle By Name(cluster=w311, "Class.Icon"=w310) -> (w309:T1)
      n123 = call "Set Undo Flag.vi"("error in"=w307, "Data in"=w309) -> ("error out"=w306:errorcluster, "Data out"=w308:T1)  [unwired: 8 in]
    }
    frame "Redo", "Undo" {
      w339 = FALSE ("TM Set?")
      n124 = Unbundle By Name(w333) -> ("Class.Ants"=w332:refnum<class "Ants.lvclass">, "Ref.TextMarker"=w337:refnum<vi>)
      n125 = Equal?(x=w335, y="Undo") -> (x = y?=w328:bool)
      n126 = call "FireAntsEvent.vi"("error in (no error)"=w331, "Ants in"=w332) -> ("error out"=w329:errorcluster)  [unwired: 2 in, 7 out]
      n127 = property class="Str"(reference=w337, "Visible"=FALSE) -> ()  [unwired: 1 in, 2 out]
      n128 = call "Const Temp Coordinate 4 points.vi"() -> ("Const Temp Coordinate"=w341:T22)  [unwired: 11 out]
      n129 = call "Const Temp Coordinate 2 points.vi"() -> ("Const Temp Coordinate"=w340:T5)  [unwired: 11 out]
      n130 = call "Empty Picture"() -> ("empty picture"=w338:picture)
      n131 = Bundle By Name(cluster=w333, "Support.Temp Icon"=w338, "Support.CTRL Pressed"=w339, "Support.Move Selection?"=w339, "Support.TM Set?"=w339, "Support.AntsRect"=w341, "Support.AntsRect Orig"=w341, "Support.Mouse Down Coords"=w340, "Support.Temp Coord"=w340) -> (w327:T1)
      n132 = in-place {
        in-place-border: w329 -> [w348]
        in-place-border: w328 -> [w343]
        in-place-border: [w345] -> w321
        in-place-border: [w344] -> w323
        n133 = in-place-cluster #1(w327) -> ("Class.History"=w347:refnum<class "History.lvclass">)
        n134 = case shown="False" w343 {
          tunnel: w348 -> [w350 w358]
          tunnel: w347 -> [w353 w357]
          tunnel: [w352 w356] -> w346
          tunnel: [w351 w355] -> w345
          tunnel: [w349 w354] -> w344
          frame False {
            # "Redo was called"
            n135 = call "Redo.vi"("error in"=w350, "History in"=w353) -> ("error out"=w351:errorcluster, "State"=w349:string, "History out"=w352:refnum<class "History.lvclass">)  [unwired: 7 in]
          }
          frame True {
            # "Undo was called"
            n136 = call "Undo.vi"("error in"=w358, "History in"=w357) -> ("error out"=w355:errorcluster, "State"=w354:string, "History out"=w356:refnum<class "History.lvclass">)  [unwired: 7 in]
          }
        }
        n137 = in-place-cluster #1("Class.History"=w346) -> (w326:T1)
      }
      n138 = Unflatten From String(type=T12 {"Template"="", "Layers"="", "Body Text"="", "Icon Text Layer"="", "Template Layer"="", "Templates Search"="", "Glyphs Search"=""} ("State"), binary string=w323, error in (no error)=w321) -> (value=w322:T12, error out=w324:errorcluster)  [unwired: 2 in, 1 out]
      n139 = case shown="Error" w324 {
        selector: w324 -> [w362 _]
        tunnel: [w363 _] -> w342
        tunnel: w326 -> [w361 w364]
        tunnel: [w360 w364] -> w330
        tunnel: w322 -> [w359 _]
        frame No Error {
          # "Set the state of editor."
          n140 = call "Set to State.vi"("error in"=w362, "State"=w359, "Data in"=w361) -> ("error out"=w363:errorcluster, "Data out"=w360:T1)  [unwired: 5 in, 2 out]
        }
        frame Error {
          # "Only likely error is\nan invalid state"
          # "Do not propagate error."
        }
      }
      n141 = Merge Errors(w321, w342) -> (w320:errorcluster)
    }
    frame "Select All" {
      n142 = Unbundle By Name(w370) -> ("Ref.Search Templates"=w369:refnum<vi>, "Ref.Line Text"=w368:refnum<vi>[], "Ref.Search Glyphs"=w367:refnum<vi>, "Ref.LayerNames"=w366:refnum<vi>[])
      n143 = Build Array (concatenate)(w369, w368, w367, w366) -> (w365:refnum<vi>[])
      n144 = for {
        tunnel: w365 -> [w406] mode=indexing
        tunnel: [w405] -> w371
        tunnel: [w404] -> w372
        stop <- w404 stop-if-true
        n145 = property class="Str"(reference=w406) -> (reference out=w405:refnum<vi>, "Key Focus"=w404:bool)  [unwired: 1 in, 1 out]
      }
      n146 = case shown="False" w372 {
        tunnel: w375 -> [w395 w399]
        tunnel: w370 -> [w380 w400]
        tunnel: [w382 w400] -> w374
        tunnel: [w381 w402] -> w373
        tunnel: w371 -> [_ w403]
        frame False {
          w397 = T23 {"Left"=0, "Top"=0, "Right"=32, "Bottom"=32} ("Rectangle")
          # "String control does not have focus"
          n147 = Unbundle By Name(w380) -> ("Class.Icon"=w379:refnum<class "Icon.lvclass">, "Class.Ants"=w378:refnum<class "Ants.lvclass">, "Ref.Tools"=w377:refnum<vi>, "Ref.Ants"=w376:refnum<vi>)
          n148 = property class="Pict"(reference=w376, error in=w395, "Visible"=TRUE) -> (error out=w390:errorcluster)  [unwired: 1 out]
          n149 = property class="RadioBtnsControl (strict)"(reference=w377, error in=w390, "Value"=T13."Select" ("Value (Signaling)")) -> (error out=w391:errorcluster)  [unwired: 1 out]
          n150 = call "Const Temp Coordinate 2 points.vi"() -> ("Const Temp Coordinate"=w394:T5)  [unwired: 11 out]
          n151 = Bundle By Name(cluster=w380, "Support.CTRL Pressed"=FALSE, "Support.Tool (old value)"=u32 111, "Support.Mouse Move Coords"=w394, "Support.Mouse Down Coords"=w394, "Support.AntsRect"=w397, "Support.AntsRect Orig"=w397) -> (w383:T1)
          n152 = call "FireAntsEvent.vi"("error in (no error)"=w391, "Rectangle (default: deselect)"=w397, "Ants in"=w378) -> ("error out"=w388:errorcluster)  [unwired: 1 in, 7 out]
          n153 = call-dynamic "GET_All User Layers.vi"("error in (no error)"=w388, "Icon.lvclass in"=w379) -> ("error out"=w384:errorcluster, "User Layer"=w387:refnum<class "Layer.lvclass">[])  [unwired: 7 in, 1 out]
          n154 = Array Size(array=w387) -> (size(s)=w386:i32)
          n155 = for {
            N: w386 -> [_]
            tunnel: [w398] -> w385 mode=indexing
            i -> [w398]
          }
          n156 = call "Set active Layer programmatically.vi"("error in"=w384, "Active Layer []"=w385, "Data in"=w383) -> ("error out"=w381:errorcluster, "Data out"=w382:T1)  [unwired: 7 in]
        }
        frame True {
          # "Text Control is being edited. Select all text inside that control."
          n157 = property class="Str"(reference=w403, error in=w399, "Text.Selection"=T14 {"Selection Start"=0, "Selection End"=4294967295}) -> (error out=w402:errorcluster)  [unwired: 1 out]
        }
      }
    }
    frame "Select Font", "Settings" {
      n158 = Equal?(x=w416, y="Select Font") -> (x = y?=w414:bool)
      n159 = Select(t="Text" ("y"), s=w414, f="") -> (s? t:f=w411:string)
      n160 = call "IconEditorSettings.vi"("error in (no error)"=w407, "Active Tag"=w411, "Data in"=w410) -> ("error out"=w409:errorcluster, "Data out"=w408:T1)  [unwired: 7 out]
    }
    frame "Select None" {
      n161 = call "Escape.vi"("error in"=w424, "Data in"=w423) -> ("error out"=w419:errorcluster, "Data out"=w420:T1)  [unwired: 2 in, 6 out]
      n162 = call "DeselectLayer.vi"("error in (no error)"=w419, "Data in"=w420) -> ("error out"=w422:errorcluster, "Data out"=w421:T1)  [unwired: 8 out]
      n163 = call "Reset layer template selection.vi"("error in (no error)"=w422, "Data in"=w421) -> ("error out"=w418:errorcluster, "Data out"=w417:T1)  [unwired: 1 in, 7 out]
    }
    frame "Show Terminals" {
      n164 = Unbundle By Name(w430) -> ("Class.Settings"=w431:refnum<class "Settings.lvclass">)
      n165 = call-dynamic "GET_Show.vi"("error in"=w426, "Settings.lvclass in"=w431) -> ("error out"=w436:errorcluster, "Show Terminals?"=w433:bool, "Settings.lvclass out"=w438:refnum<class "Settings.lvclass">)  [unwired: 7 out]
      n166 = Not(x=w433) -> (.not. x?=w434:bool)
      n167 = call "ShowTerminals.vi"("Set Pic? (T)"=TRUE, "error in"=w436, "Tag enabled?"=TRUE, "Show Terminals?"=w434, "Data in"=w430) -> ("error out"=w435:errorcluster, "Data out"=w429:T1)  [unwired: 1 in, 4 out]
      n168 = call-dynamic "SET_Show.vi"("error in"=w435, "Show Terminals?"=w434, "Settings.lvclass in"=w438) -> ("error out"=w427:errorcluster, "Settings.lvclass out"=w428:refnum<class "Settings.lvclass">)  [unwired: 1 in, 6 out]
      n169 = Bundle By Name(cluster=w429, "Class.Settings"=w428) -> (w425:T1)
    }
    frame "Synchronize with Icon Library" {
      n170 = vi-ref "ni.com_iconlibrary.vi"() -> (w450:refnum<vi>)
      n171 = property class="VI"(reference=w450, error in=w448) -> (error out=w447:errorcluster, "Path"=w449:path)  [unwired: 1 out]
      n172 = Open VI Reference(vi path=w449, error in (no error)=w447) -> (vi reference=w451:refnum<vi>, error out=w452:errorcluster)  [unwired: 4 in]
      n173 = invoke class="VI" method="Run VI"(reference=w451, error in=w452, "Wait until done"=TRUE ("Wait Until Done"), "Auto Dispose Ref"=FALSE ("Auto Dispose Reference")) -> (reference out=w443:refnum<vi>, error out=w444:errorcluster)  [unwired: 1 in, 3 out]
      n174 = Close Reference(reference=w443, error in (no error)=w444) -> (error out=w441:errorcluster)
      n175 = Unbundle By Name(w441) -> ("code"=w442:i32)
      n176 = case shown="0, Default" w442 {
        tunnel: [w460 errorcluster {"status"=FALSE, "code"=0, "source"=""} ("error out")] -> w454
        tunnel: w453 -> [w459 _]
        tunnel: w441 -> [w458 _]
        tunnel: w440 -> [w457 w462]
        tunnel: [w457 w462] -> w439
        frame 0, Default {
          n177 = Unbundle By Name(w457) -> ("Ref.GlyphLoadAnimation"=w455:refnum<vi>, "Ref.refreshGlyphs"=w456:refnum<vi>)
          n178 = call "Launch Dynamically Load Graphics.vi"("User events"=w459, "Path"=Pathes."Glyphs", "error in (no error)"=w458, "button ref"=w456, "animatedDecoration ref"=w455) -> ("error out"=w460:errorcluster)  [unwired: 1 in, 5 out]
        }
        frame 1039 {
          # "VI was aborted"
        }
      }
    }
    frame "Template" {
      n179 = call "DrawIcon.vi"("Tools"=Tools."Ellipse", "error in (no error)"=w470, "Data in"=w475) -> ("error out"=w481:errorcluster, "Icon"=w480:picture, "Data out"=w466:T1)  [unwired: 2 in, 4 out]
      n180 = call "Read Data from Caller.vi"() -> ("Icon Editor Invoker Type"=w477:T24)  [unwired: 3 in, 8 out]
      n181 = call "Specify Path Enum.vi"("Icon Editor Invoker Type"=w477) -> ("Path"=w476:T9)  [unwired: 10 out]
      n182 = call "Get LV Glyph Path.vi"("Path"=w476, "error in (no error)"=w481) -> ("error out"=w474:errorcluster, "Requested Path"=w471:path)  [unwired: 1 in, 7 out]
      n183 = call "Get Image Data.vi"("Pic In"=w480) -> ("image data out"=w479:T16)  [unwired: 3 in, 7 out]
      n184 = call "Save Graphic.vi"("Loc string caption"=w467, "FP Title"=w472, "error in (no error)"=w474, "Start path in"=w471) -> ("error out"=w473:errorcluster, "Output"=w464:path)  [unwired: 6 out]
      n185 = Empty String/Path?(string/path=w464) -> (empty?=w468:bool)
      n186 = case shown="False" w468 {
        tunnel: w479 -> [w494 _]
        tunnel: w478 -> [w491 _]
        tunnel: w476 -> [w485 _]
        tunnel: w473 -> [w490 w498]
        tunnel: w464 -> [w484 _]
        tunnel: [w489 w498] -> w469
        tunnel: w466 -> [w488 w497]
        tunnel: [w488 w497] -> w465
        frame False {
          n187 = flat-sequence {
            tunnel: w484 -> [w496]
            tunnel: [w496] -> w483
            frame #0 {
              # "If the user pathologically deleted the specified folder while the dialog was up, this code will ensure that the owning folder exists when trying to save the .png file."
              n188 = Strip Path(path=w496) -> (stripped path=w495:path)  [unwired: 1 out]
              n189 = call <vilib>:"Create Directory Recursive.vi"("directory"=w495) -> ()  [unwired: 4 in, 3 out]
            }
          }
          n190 = Unbundle By Name(w488) -> ("Ref.TemplateLoadAnimation"=w487:refnum<vi>, "Ref.refreshTemplates"=w486:refnum<vi>)
          n191 = call <vilib>:"Write PNG File.vi"("error in (no error)"=w490, "image data"=w494, "path to PNG file"=w483) -> ("error out"=w493:errorcluster)  [unwired: 1 in, 7 out]
          n192 = call "Launch Dynamically Load Graphics.vi"("User events"=w491, "Template saved?"=TRUE, "Path"=w485, "error in (no error)"=w493, "button ref"=w486, "animatedDecoration ref"=w487) -> ("error out"=w489:errorcluster)  [unwired: 5 out]
        }
        frame True {
        }
      }
    }
    frame "Show Block Diagram" {
      n193 = property class="VI"(reference=w503, error in=w500, "BDWin.Open"=TRUE ("Block Diagram Window:Open")) -> (error out=w501:errorcluster)  [unwired: 1 out]
    }
    frame Default {
    }
  }
  n194 = call "ViewLayer.vi"("error in (no error)"=w15, "Data in"=w13) -> ("error out"=w7:errorcluster, "Data out"=→"Data out":T1)  [unwired: 2 in, 6 out]
  n195 = call "Defer_FP_Updates.vi"("Defer Panel Updates"=FALSE, "error in"=w7, "lv_icon.vi in"=w5) -> ("error out"=→"error out":errorcluster)  [unwired: 8 out]
